vi "Configure Marker Frequency.vi"(8 "error in (no error)":errorcluster, 9 "Marker Number (1)":u32=1 min=1, 10 "Marker Frequency [Hz]":dbl, 11 "SA-FSW in":refnum<class "SA-FSW.lvclass">) -> (0 "error out":errorcluster, 3 "SA-FSW out":refnum<class "SA-FSW.lvclass">)   [LabVIEW 2020, in "SA-FSW.lvclass"]
uses:
  SA-FSW.lvclass
  C:/Sandbox/Git_Sandbox/WiSpry Test Framework source code (LV20)/WiSpry Test Framework/Instruments/Instrument.lvclass
  Instrument.lvclass/Instrument.ctl
  Instrument.lvclass
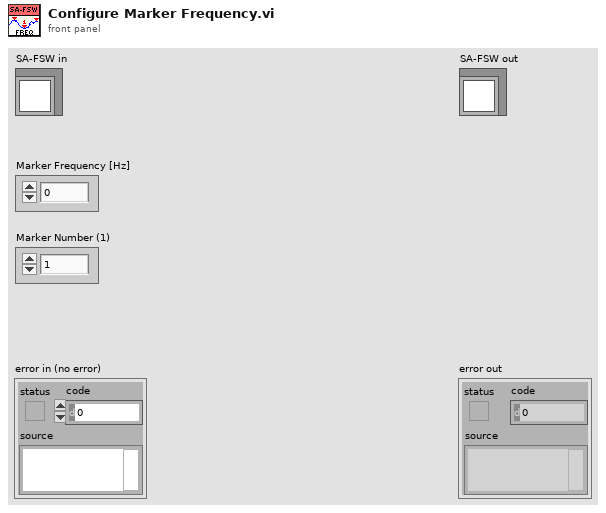
[diagram p1: front panel]
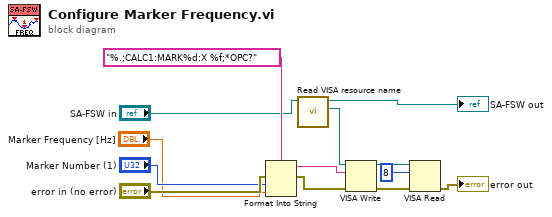
[diagram p0: block diagram]
diagram:
  n1 = Format Into String(format string="%.;CALC1:MARK%d:X %f;*OPC?", error in="error in (no error)", "Marker Number (1)", "Marker Frequency [Hz]") -> (resulting string=w7:string, error out=w6:errorcluster)  [unwired: 1 in]
  n2 = call "Read VISA resource name.vi"("Instrument in"="SA-FSW in") -> ("VISA resource name"=w8:refnum<visa-resource-name>, "Instrument out"=→"SA-FSW out":refnum<class "SA-FSW.lvclass">)  [unwired: 9 in]
  n3 = VISA Write(VISA resource name=w8, write buffer=w7, error in (no error)=w6) -> (VISA resource name out=w3:refnum<visa-resource-name>, error out=w4:errorcluster)  [unwired: 1 out]
  n4 = VISA Read(VISA resource name=w3, byte count=u32 8, error in (no error)=w4) -> (error out=→"error out":errorcluster)  [unwired: 3 out]
